vi "SW_Gen_Draw_Segments.vi"(6 "Colors cluster":T3, 7 "Show magnets":bool, 8 "Cluster of image geometrical and scaling parameters":T1, 9 "Input cluster of parameters":T4={"Amount of border segments"=8, "Border segments starting angle"=0, "Amount of midfield segments"=4, "Midfield segments starting angle"=0, "Midfield segments outer radius, mm"=60, "Amount of central segments"=1, "Center segment outer radius, mm"=30, "Diameter of the cage, mm"=180, "R-gap between segments, mm"=10} {"Diameter of the cage, mm" scale=20.0..250.0}, 10 "Bounding rectangles":T2, 11 "Zones display background in":picture) -> (1 "Array of the pixel to color correspondences":u32[][](array[numeric]), 2 "No zones image":picture, 3 "Zones in the cage layout":picture)   [LabVIEW 2016]
panel:
  in  "Color of the South magnet":u32(colorbox)=16711680
  in  "Color of the North magnet":u32(colorbox)=9567230
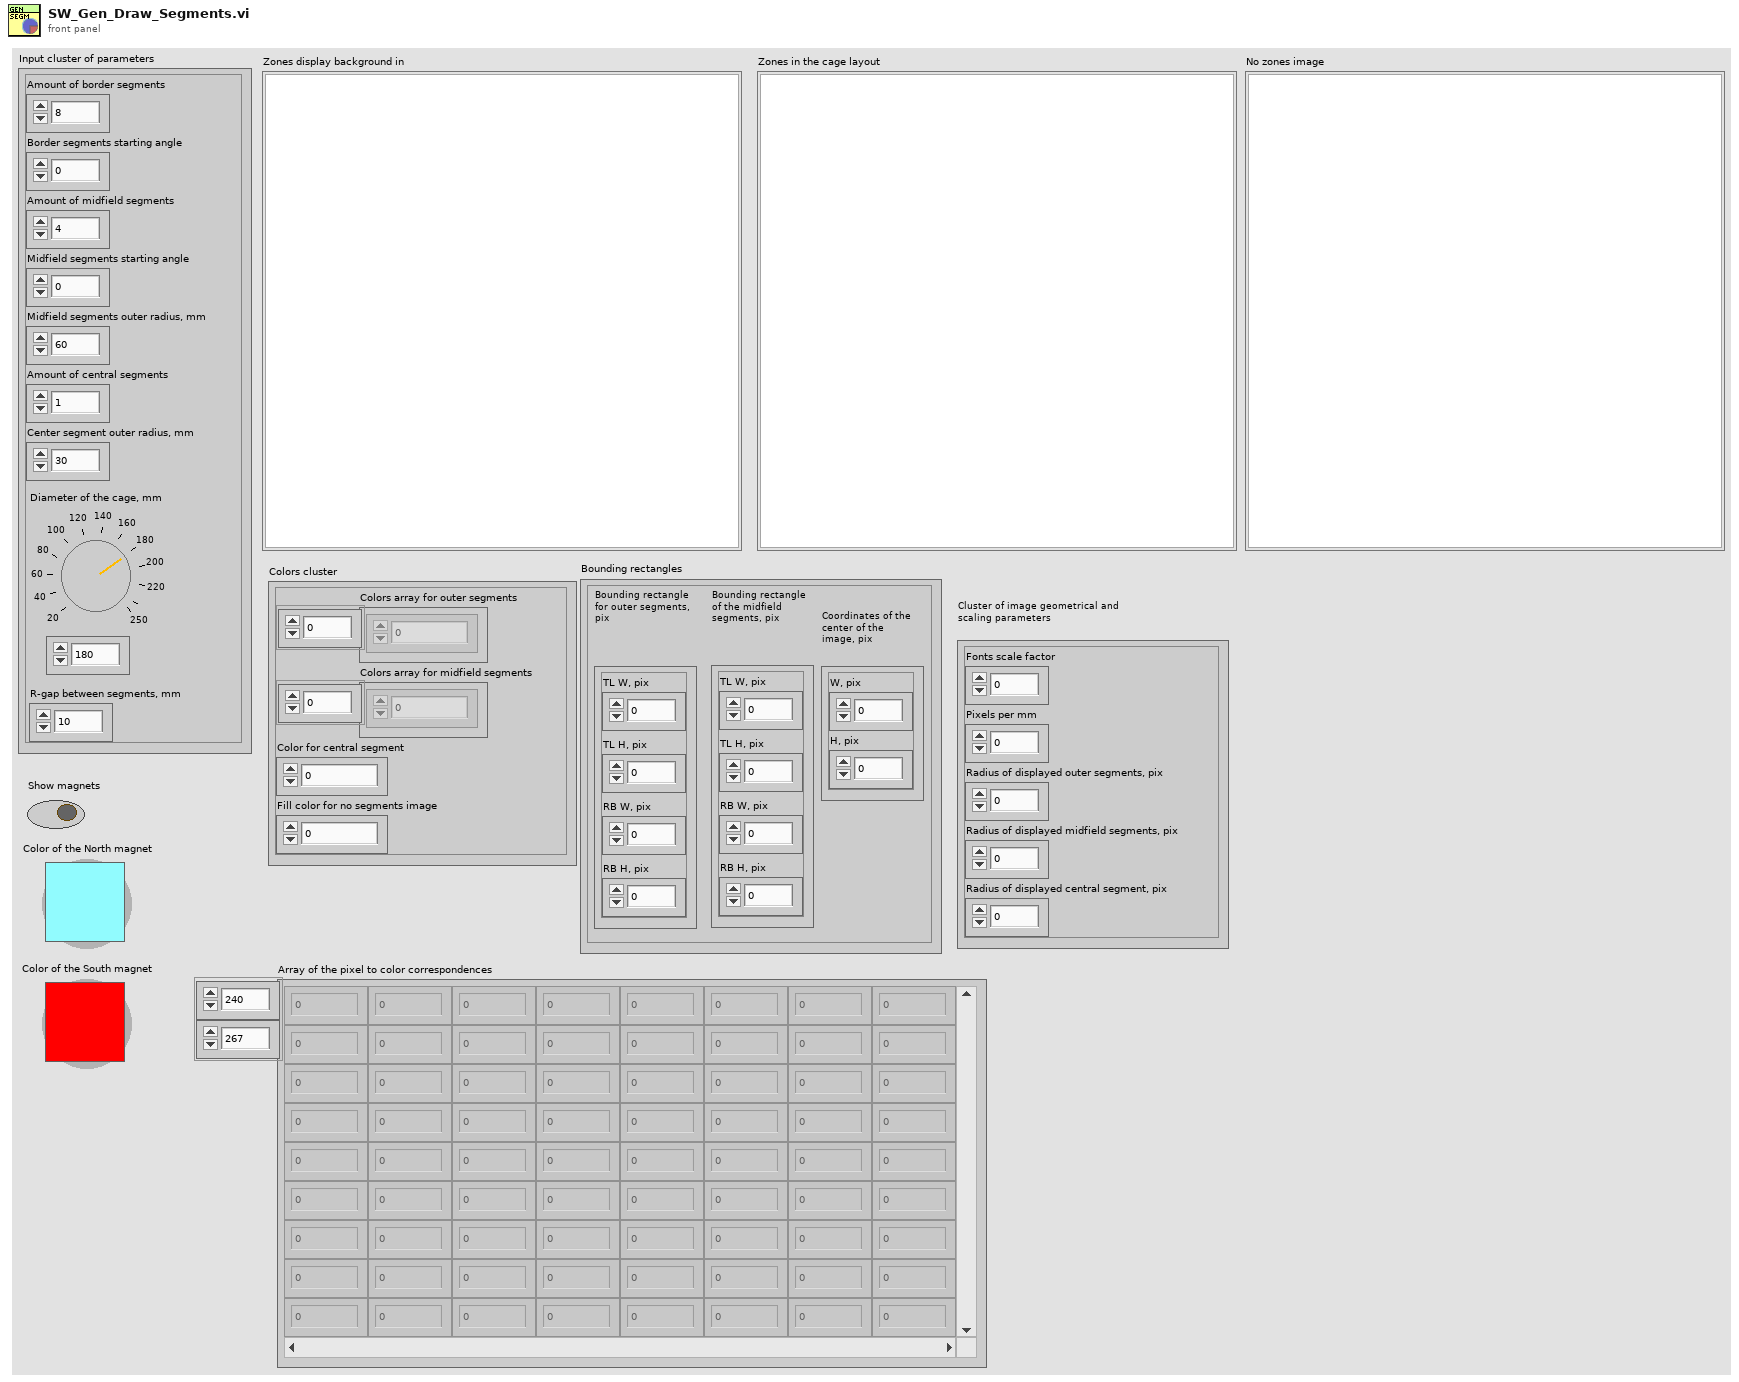
[diagram p1: front panel]
types:
  T1 = cluster{"Fonts scale factor":dbl, "Pixels per mm":dbl, "Radius of displayed outer segments, pix":dbl, "Radius of displayed midfield segments, pix":dbl, "Radius of displayed central segment, pix":dbl}
  T2 = cluster{"Bounding rectangle for outer segments, pix":cluster{"TL W, pix":dbl, "TL H, pix":dbl, "RB W, pix":dbl, "RB H, pix":dbl}, "Bounding rectangle of the midfield segments, pix":cluster{"TL W, pix":dbl, "TL H, pix":dbl, "RB W, pix":dbl, "RB H, pix":dbl}, "Coordinates of the center of the image, pix":cluster{"W, pix":dbl, "H, pix":dbl}}
  T3 = cluster{"Colors array for outer segments":u32[], "Colors array for midfield segments":u32[], "Color for central segment":u32, "Fill color for no segments image":u32}
  T4 = cluster{"Amount of border segments":u8, "Border segments starting angle":i16, "Amount of midfield segments":u8, "Midfield segments starting angle":i16, "Midfield segments outer radius, mm":u16, "Amount of central segments":u8, "Center segment outer radius, mm":u16, "Diameter of the cage, mm":u16, "R-gap between segments, mm":u8}
  T5 = cluster{"Width":u16, "Style":enum32{"Solid", "Dash", "Dot", "DashDot", "DashDotDot"}}
  T6 = cluster{"TL W, pix":dbl, "TL H, pix":dbl, "RB W, pix":dbl, "RB H, pix":dbl}
  T7 = typedef "imagedata.ctl" = cluster{"image type":i32, "image depth":i32, "image":u8[], "mask":u8[], "colors":u32[], "Rectangle":cluster{"left":i16, "top":i16, "right":i16, "bottom":i16}}
  T8 = cluster{"left":i16, "top":i16, "right":i16, "bottom":i16}
  T9 = cluster{"image[0]":u8, "image[1]":u8, "image[2]":u8}
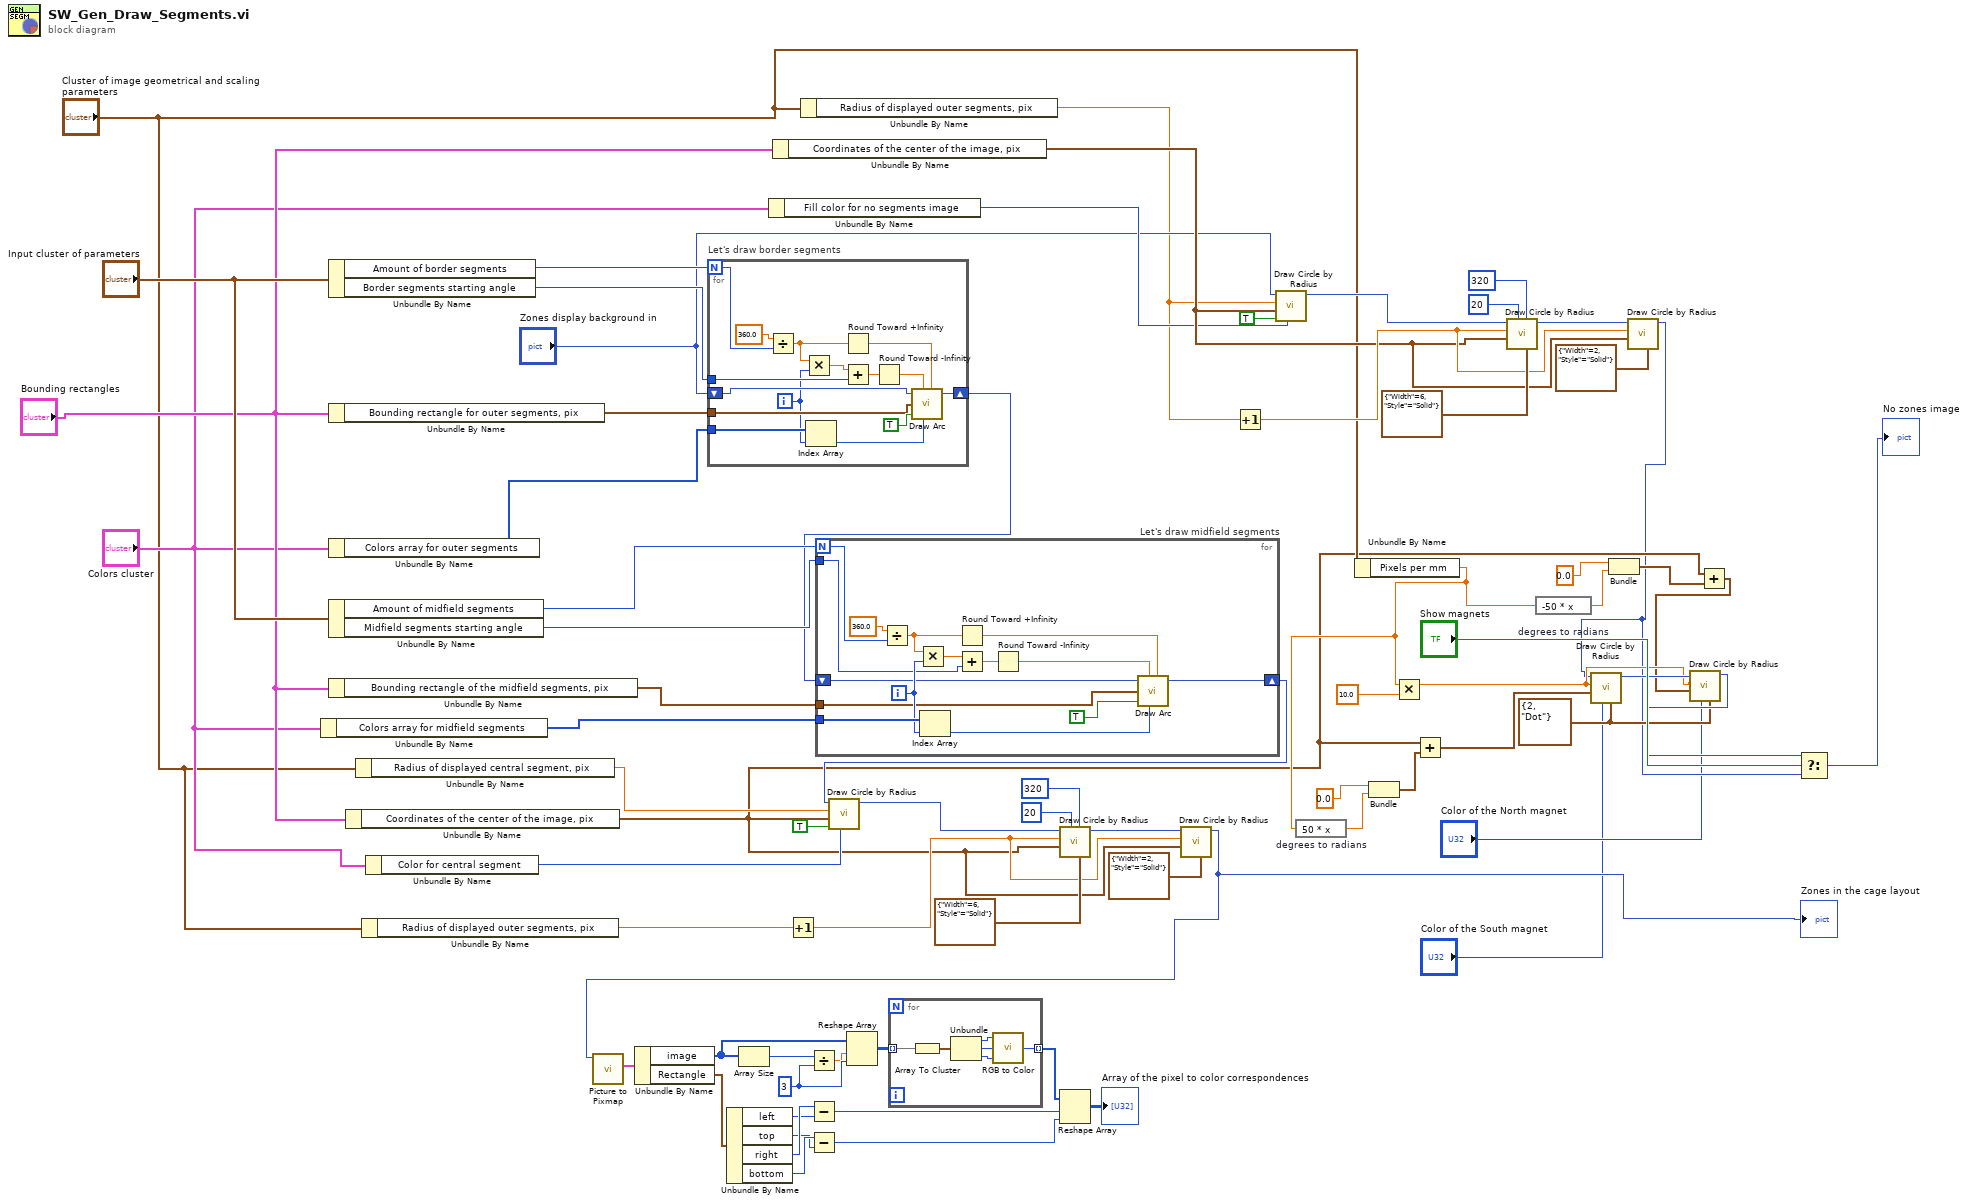
[diagram p0: block diagram]
diagram:
  w14 = T5 {"Width"=2, "Style"=enum."Dot"} ("pen")
  w49 = 3 ("dimension size")
  n1 = Unbundle By Name("Colors cluster") -> ("Colors array for midfield segments"=w65:u32[])
  n2 = Unbundle By Name("Input cluster of parameters") -> ("Amount of border segments"=w73:u8, "Border segments starting angle"=w72:i16)
  n3 = Unbundle By Name("Bounding rectangles") -> ("Bounding rectangle for outer segments, pix"=w71:T6)
  n4 = Unbundle By Name("Colors cluster") -> ("Colors array for outer segments"=w70:u32[])
  n5 = Unbundle By Name("Input cluster of parameters") -> ("Amount of midfield segments"=w69:u8, "Midfield segments starting angle"=w68:i16)
  n6 = Unbundle By Name("Bounding rectangles") -> ("Bounding rectangle of the midfield segments, pix"=w66:T6)
  n7 = Unbundle By Name("Bounding rectangles") -> ("Coordinates of the center of the image, pix"=w8:cluster{"W, pix":dbl, "H, pix":dbl})
  n8 = Unbundle By Name("Cluster of image geometrical and scaling parameters") -> ("Radius of displayed central segment, pix"=w24:dbl)
  n9 = Unbundle By Name("Cluster of image geometrical and scaling parameters") -> ("Radius of displayed outer segments, pix"=w54:dbl)
  n10 = Unbundle By Name("Colors cluster") -> ("Color for central segment"=w63:u32)
  n11 = for "Let's draw border segments" {
    N: w73 -> [w80]
    tunnel: w72 -> [w85]
    shift-right: [w78] -> w67
    shift-left: "Zones display background in" -> [w87]
    tunnel: w71 -> [w81]
    tunnel: w70 -> [w84]
    i -> [w75]
    n12 = Divide(x=360.0, y=w80) -> (x/y=w79:dbl)
    n13 = Multiply(x=w79, y=w75) -> (x*y=w86:dbl)
    n14 = Index Array(array=w84, index=w75) -> (element=w74:u32)
    n15 = Round Toward +Infinity(x=w79) -> (ceil(x): smallest int >= x=w77:dbl)
    n16 = Add(x=w86, y=w85) -> (x+y=w82:dbl)
    n17 = Round Toward -Infinity(1:w82) -> (0:w76:dbl)
    n18 = call <vilib>:"Draw Arc.vi"("picture"=w87, "start angle[degrees]"=w76, "rect"=w81, "fill?(F)"=TRUE, "color(black)"=w74, "arc size[degrees]"=w77) -> ("new picture"=w78:picture)  [unwired: 3 in]
  }
  n19 = Unbundle By Name("Colors cluster") -> ("Fill color for no segments image"=w26:u32)
  n20 = Unbundle By Name("Bounding rectangles") -> ("Coordinates of the center of the image, pix"=w28:cluster{"W, pix":dbl, "H, pix":dbl})
  n21 = Increment(x=w54) -> (x+1=w53:dbl)
  n22 = Unbundle By Name("Cluster of image geometrical and scaling parameters") -> ("Radius of displayed outer segments, pix"=w21:dbl)
  n23 = for "Let's draw midfield segments" {
    N: w69 -> [w94]
    shift-right: [w89] -> w64
    shift-left: w67 -> [w90]
    tunnel: w68 -> [w92]
    tunnel: w66 -> [w91]
    tunnel: w65 -> [w96]
    i -> [w93]
    n24 = Divide(x=360.0, y=w94) -> (x/y=w98:dbl)
    n25 = Multiply(x=w98, y=w93) -> (x*y=w99:dbl)
    n26 = Index Array(array=w96, index=w93) -> (element=w95:u32)
    n27 = Round Toward +Infinity(x=w98) -> (ceil(x): smallest int >= x=w101:dbl)
    n28 = Add(x=w99, y=w92) -> (x+y=w100:dbl)
    n29 = Round Toward -Infinity(1:w100) -> (0:w102:dbl)
    n30 = call <vilib>:"Draw Arc.vi"("picture"=w90, "start angle[degrees]"=w102, "rect"=w91, "fill?(F)"=TRUE, "color(black)"=w95, "arc size[degrees]"=w101) -> ("new picture"=w89:picture)  [unwired: 3 in]
  }
  n31 = call <vilib>:"Draw Circle by Radius.vi"("color(black)"=w63, "fill?(F)"=TRUE, "pixel center"=w8, "radius"=w24, "picture"=w64) -> ("new picture"=w55:picture)  [unwired: 6 in]
  n32 = call <vilib>:"Draw Circle by Radius.vi"("pen"=T5 {"Width"=6, "Style"=enum."Solid"}, "arc size(360)"=i16 320, "start angle(0)"=i16 20, "pixel center"=w8, "radius"=w53, "picture"=w55) -> ("new picture"=w60:picture)  [unwired: 5 in]
  n33 = call <vilib>:"Draw Circle by Radius.vi"("pen"=T5 {"Width"=2, "Style"=enum."Solid"}, "pixel center"=w8, "radius"=w53, "picture"=w60) -> ("new picture"=w5:picture)  [unwired: 7 in]
  "Zones in the cage layout" <- w5
  n34 = call <vilib>:"Picture to Pixmap.vi"("picture"=w5) -> ("image data"=w52:T7)  [unwired: 9 in, 1 out]
  n35 = Unbundle By Name(w52) -> ("image"=w51:u8[], "Rectangle"=w46:T8)
  n36 = Unbundle By Name(w46) -> ("left"=w43:i16, "top"=w40:i16, "right"=w44:i16, "bottom"=w41:i16)
  n37 = Array Size(array=w51) -> (size(s)=w50:i32)
  n38 = Divide(x=w50, y=w49) -> (x/y=w48:dbl)
  n39 = Subtract(x=w44, y=w43) -> (x-y=w42:i16)
  n40 = Subtract(x=w41, y=w40) -> (x-y=w39:i16)
  n41 = Reshape Array(w51, w48, w49) -> (w47:u8[][])
  n42 = for {
    tunnel: w47 -> [w109] mode=indexing
    tunnel: [w104] -> w45 mode=indexing
    n43 = Array To Cluster(array=w109) -> (cluster=w108:T9)
    n44 = Unbundle(w108) -> ("image[0]"=w107:u8, "image[1]"=w106:u8, "image[2]"=w105:u8)
    n45 = call <vilib>:"RGB to Color.vi"("B"=w105, "G"=w106, "R"=w107) -> ("Color"=w104:u32)
  }
  n46 = Reshape Array(w45, w42, w39) -> (→"Array of the pixel to color correspondences":u32[][])
  n47 = Increment(x=w21) -> (x+1=w30:dbl)
  n48 = call <vilib>:"Draw Circle by Radius.vi"("color(black)"=w26, "fill?(F)"=TRUE, "pixel center"=w28, "radius"=w21, "picture"="Zones display background in") -> ("new picture"=w31:picture)  [unwired: 6 in]
  n49 = Unbundle By Name("Cluster of image geometrical and scaling parameters") -> ("Pixels per mm"=w9:dbl)
  n50 = expression code="50 * x" "degrees to radians"(w9) -> (w18:dbl)
  n51 = Bundle("W, pix"=0.0, "Pixels per mm"=w18) -> (w17:cluster{"W, pix":dbl, "Pixels per mm":dbl})  [unwired: 1 in]
  n52 = Multiply(x=w9, y=10.0) -> (x*y=w13:dbl)
  n53 = Add(x=w8, y=w17) -> (x+y=w12:cluster{"W, pix":dbl, dbl})
  n54 = call <vilib>:"Draw Circle by Radius.vi"("pen"=T5 {"Width"=6, "Style"=enum."Solid"}, "arc size(360)"=i16 320, "start angle(0)"=i16 20, "pixel center"=w28, "radius"=w30, "picture"=w31) -> ("new picture"=w36:picture)  [unwired: 5 in]
  n55 = expression code="-50 * x" "degrees to radians"(w9) -> (w10:dbl)
  n56 = Bundle("W, pix"=0.0, "Pixels per mm"=w10) -> (w7:cluster{"W, pix":dbl, "Pixels per mm":dbl})  [unwired: 1 in]
  n57 = call <vilib>:"Draw Circle by Radius.vi"("pen"=T5 {"Width"=2, "Style"=enum."Solid"}, "pixel center"=w28, "radius"=w30, "picture"=w36) -> ("new picture"=w3:picture)  [unwired: 7 in]
  n58 = call <vilib>:"Draw Circle by Radius.vi"("pen"=w14, "color(black)"="Color of the South magnet", "pixel center"=w12, "radius"=w13, "picture"=w3) -> ("new picture"=w16:picture)  [unwired: 6 in]
  n59 = Add(x=w8, y=w7) -> (x+y=w6:cluster{"W, pix":dbl, dbl})
  n60 = call <vilib>:"Draw Circle by Radius.vi"("pen"=w14, "color(black)"="Color of the North magnet", "pixel center"=w6, "radius"=w13, "picture"=w16) -> ("new picture"=w15:picture)  [unwired: 6 in]
  n61 = Select(t=w15, s="Show magnets", f=w3) -> (s? t:f=→"No zones image":picture)
